vi "Set Speaker Switch.vi"(8 "error in":errorcluster, 10 "State":bool, 11 "PAS in":refnum<class "PAS.lvclass">) -> (0 "error out":errorcluster, 3 "PAS out":refnum<class "PAS.lvclass">)   [LabVIEW 2015, in "PAS.lvclass"]
uses:
  PAS.lvclass
  PAS.lvclass/PAS.ctl
  Switch/Switch.lvclass
  Data/Main/PAS Data.lvclass
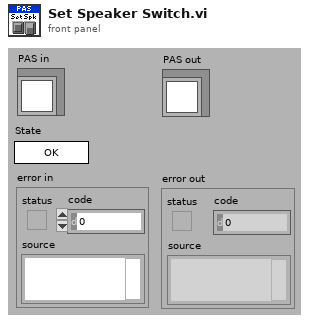
[diagram p1: front panel]
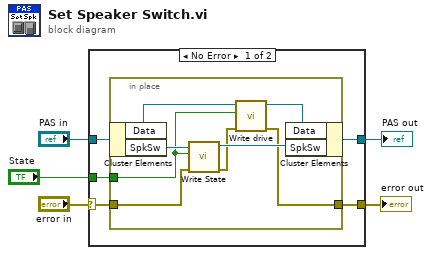
[diagram p0: block diagram]
diagram:
  n1 = case shown="No Error" "error in" {
    selector: "error in" -> [w8 w20]
    tunnel: [w7 w20] -> w4
    tunnel: [w9 w19] -> w2
    tunnel: "PAS in" -> [w10 w19]
    tunnel: "State" -> [w6 _]
    frame No Error {
      n2 = in-place {
        in-place-border: w8 -> [w16]
        in-place-border: [w13] -> w7
        in-place-border: w6 -> [w12]
        n3 = in-place-cluster #1(w10) -> ("Data"=w15:refnum<class "PAS Data.lvclass">, "SpkSw"=w18:refnum<class "Switch.lvclass">)
        n4 = call-dynamic "Write State.vi"("error in"=w16, "State"=w12, "Switch in"=w18) -> ("error out"=w14:errorcluster, "Switch out"=w17:refnum<class "Switch.lvclass">)  [unwired: 7 in]
        n5 = call "Write drive.vi"("error in"=w14, "drive"=w12, "PAS Data in"=w15) -> ("error out"=w13:errorcluster, "PAS Data out"=w11:refnum<class "PAS Data.lvclass">)  [unwired: 7 in]
        n6 = in-place-cluster #1("Data"=w11, "SpkSw"=w17) -> (w9:refnum<class "PAS.lvclass">)
      }
    }
    frame Error {
    }
  }
  "error out" <- w4
  "PAS out" <- w2
